vi "1SDI_State_v00.vi"(4 "BS Hold Pulse":bool, 6 "\"I too high?\"":T6, 11 "Control Cavity Cluster":T11={"Control EPR"={"Lock"=FALSE, "Hold"=FALSE, "P Gain"=0, "P BS"=-5, "I Gain"=0, "I BS"=-10, "I2 G"=0, "I2 BS"=-26, "Scan Amp"=0, "Scan Off"=0, "Scan FS"=0, "SFS BS"=0, "I Max value"=10000, "I2 Max value"=10000, "Scope.Offset"=0, "Trigger Direction"=enum."either", "Scan-PII thresh"=0}, "Control HD A"={"Lock"=FALSE, "Hold"=FALSE, "P Gain"=0, "P BS"=-5, "I Gain"=0, "I BS"=-10, "I2 G"=0, "I2 BS"=-26, "Scan Amp"=0, "Scan Off"=0, "Scan FS"=0, "SFS BS"=0, "I Max value"=10000, "I2 Max value"=10000, "Scope.Offset"=0, "Trigger Direction"=enum."either", "Scan-PII thresh"=0}, "Control HD B"={"Lock"=FALSE, "Hold"=FALSE, "P Gain"=0, "P BS"=-5, "I Gain"=0, "I BS"=-10, "I2 G"=0, "I2 BS"=-26, "Scan Amp"=0, "Scan Off"=0, "Scan FS"=0, "SFS BS"=0, "I Max value"=10000, "I2 Max value"=10000, "Scope.Offset"=0, "Trigger Direction"=enum."either", "Scan-PII thresh"=0}, "Max"={"Max EPR"=0, "Max HD A"=0, "Max HD B"=0}, "Min"={"Min EPR"=0, "Min HD A"=0, "Min HD B"=0}, "Lock Threshold"={"EPR"=0, "HD A"=0, "HD B"=0}, "Re-Scan Threshold"={"EPR"=0, "HD A"=0, "HD B"=0}, "Lock Point?"={"EPR"=FALSE, "HD A"=FALSE, "HD B"=FALSE}, "Re-scan?"={"EPR"=FALSE, "HD A"=FALSE, "HD B"=FALSE}, "Lock pressed? (-1)"={"EPR"=FALSE, "HD A"=FALSE, "HD B"=FALSE}, "Cavity Errors"={"EPR"=0, "HD A"=0, "HD B"=0}, "State (-1)"={"EPR"=enum."Safe", "HD A"=enum."Safe", "HD B"=enum."Safe"}, "Safety First"={"lim reset"=FALSE, "no limit"=FALSE, "pos slew rate * dt"=0, "neg slew rate * dt"=0, "Hold All"=FALSE, "Count(Ticks)"=0}}) -> (3 "PII Scan State Errors":T8={"Control EPR"={"Lock"=FALSE, "Hold"=FALSE, "P Gain"=3, "P BS"=0, "I Gain"=0, "I BS"=-10, "I2 G"=0, "I2 BS"=-26, "Scan Amp"=0, "Scan Off"=0, "Scan FS"=0, "SFS BS"=0, "I Max value"=10000, "I2 Max value"=10000, "Scope.Offset"=0, "Trigger Direction"=enum."either", "Scan-PII thresh"=0}, "Control HD A"={"Lock"=FALSE, "Hold"=FALSE, "P Gain"=0, "P BS"=-5, "I Gain"=0, "I BS"=-10, "I2 G"=0, "I2 BS"=-26, "Scan Amp"=0, "Scan Off"=0, "Scan FS"=0, "SFS BS"=0, "I Max value"=10000, "I2 Max value"=10000, "Scope.Offset"=0, "Trigger Direction"=enum."either", "Scan-PII thresh"=0}, "Control HD B"={"Lock"=FALSE, "Hold"=FALSE, "P Gain"=0, "P BS"=-5, "I Gain"=0, "I BS"=-10, "I2 G"=0, "I2 BS"=-26, "Scan Amp"=0, "Scan Off"=0, "Scan FS"=0, "SFS BS"=0, "I Max value"=10000, "I2 Max value"=10000, "Scope.Offset"=0, "Trigger Direction"=enum."either", "Scan-PII thresh"=0}, "Error Signals"={"EPR"=0, "HD A"=0, "HD B"=0}, "State"={"EPR"=enum."Safe", "HD A"=enum."Safe", "HD B"=enum."Safe"}}, 5 "MaxMin":T1)   [LabVIEW 2011]
doc: "The state of the output is decided here. There are four possible states: 1) Safe - zeros; 2) Hold - constant output of last value; 3) Scan - saw tooth at low frequency 4) Lock - PII output."
uses:
  Strict Type Defs/1SDI State.ctl
  Strict Type Defs/1SDI PII Scan State.ctl
  Strict Type Defs/PII individual.ctl
  Strict Type Defs/Error Signals 1SDI.ctl
  Strict Type Defs/1SDI Lock Point.ctl
  Strict Type Defs/1SDI Control Cluster.ctl
  Strict Type Defs/1SDI Max.ctl
  Strict Type Defs/1SDI Min.ctl
  Strict Type Defs/Lock Thresh 1SDI.ctl
  Strict Type Defs/Safety First.ctl
  Strict Type Defs/1SDI MaxMin.ctl
  Strict Type Defs/1SDI Reset MaxMin.ctl
panel:
  in  "MaxMin typedef":T1
  in  "Lock?":T6
  in  "PII Scan State":T8={"Control EPR"={"Lock"=FALSE, "Hold"=FALSE, "P Gain"=3, "P BS"=0, "I Gain"=0, "I BS"=-10, "I2 G"=0, "I2 BS"=-26, "Scan Amp"=0, "Scan Off"=0, "Scan FS"=0, "SFS BS"=0, "I Max value"=10000, "I2 Max value"=10000, "Scope.Offset"=0, "Trigger Direction"=enum."either", "Scan-PII thresh"=0}, "Control HD A"={"Lock"=FALSE, "Hold"=FALSE, "P Gain"=0, "P BS"=-5, "I Gain"=0, "I BS"=-10, "I2 G"=0, "I2 BS"=-26, "Scan Amp"=0, "Scan Off"=0, "Scan FS"=0, "SFS BS"=0, "I Max value"=10000, "I2 Max value"=10000, "Scope.Offset"=0, "Trigger Direction"=enum."either", "Scan-PII thresh"=0}, "Control HD B"={"Lock"=FALSE, "Hold"=FALSE, "P Gain"=0, "P BS"=-5, "I Gain"=0, "I BS"=-10, "I2 G"=0, "I2 BS"=-26, "Scan Amp"=0, "Scan Off"=0, "Scan FS"=0, "SFS BS"=0, "I Max value"=10000, "I2 Max value"=10000, "Scope.Offset"=0, "Trigger Direction"=enum."either", "Scan-PII thresh"=0}, "Error Signals"={"EPR"=0, "HD A"=0, "HD B"=0}, "State"={"EPR"=enum."Safe", "HD A"=enum."Safe", "HD B"=enum."Safe"}}
  in  "State":T2
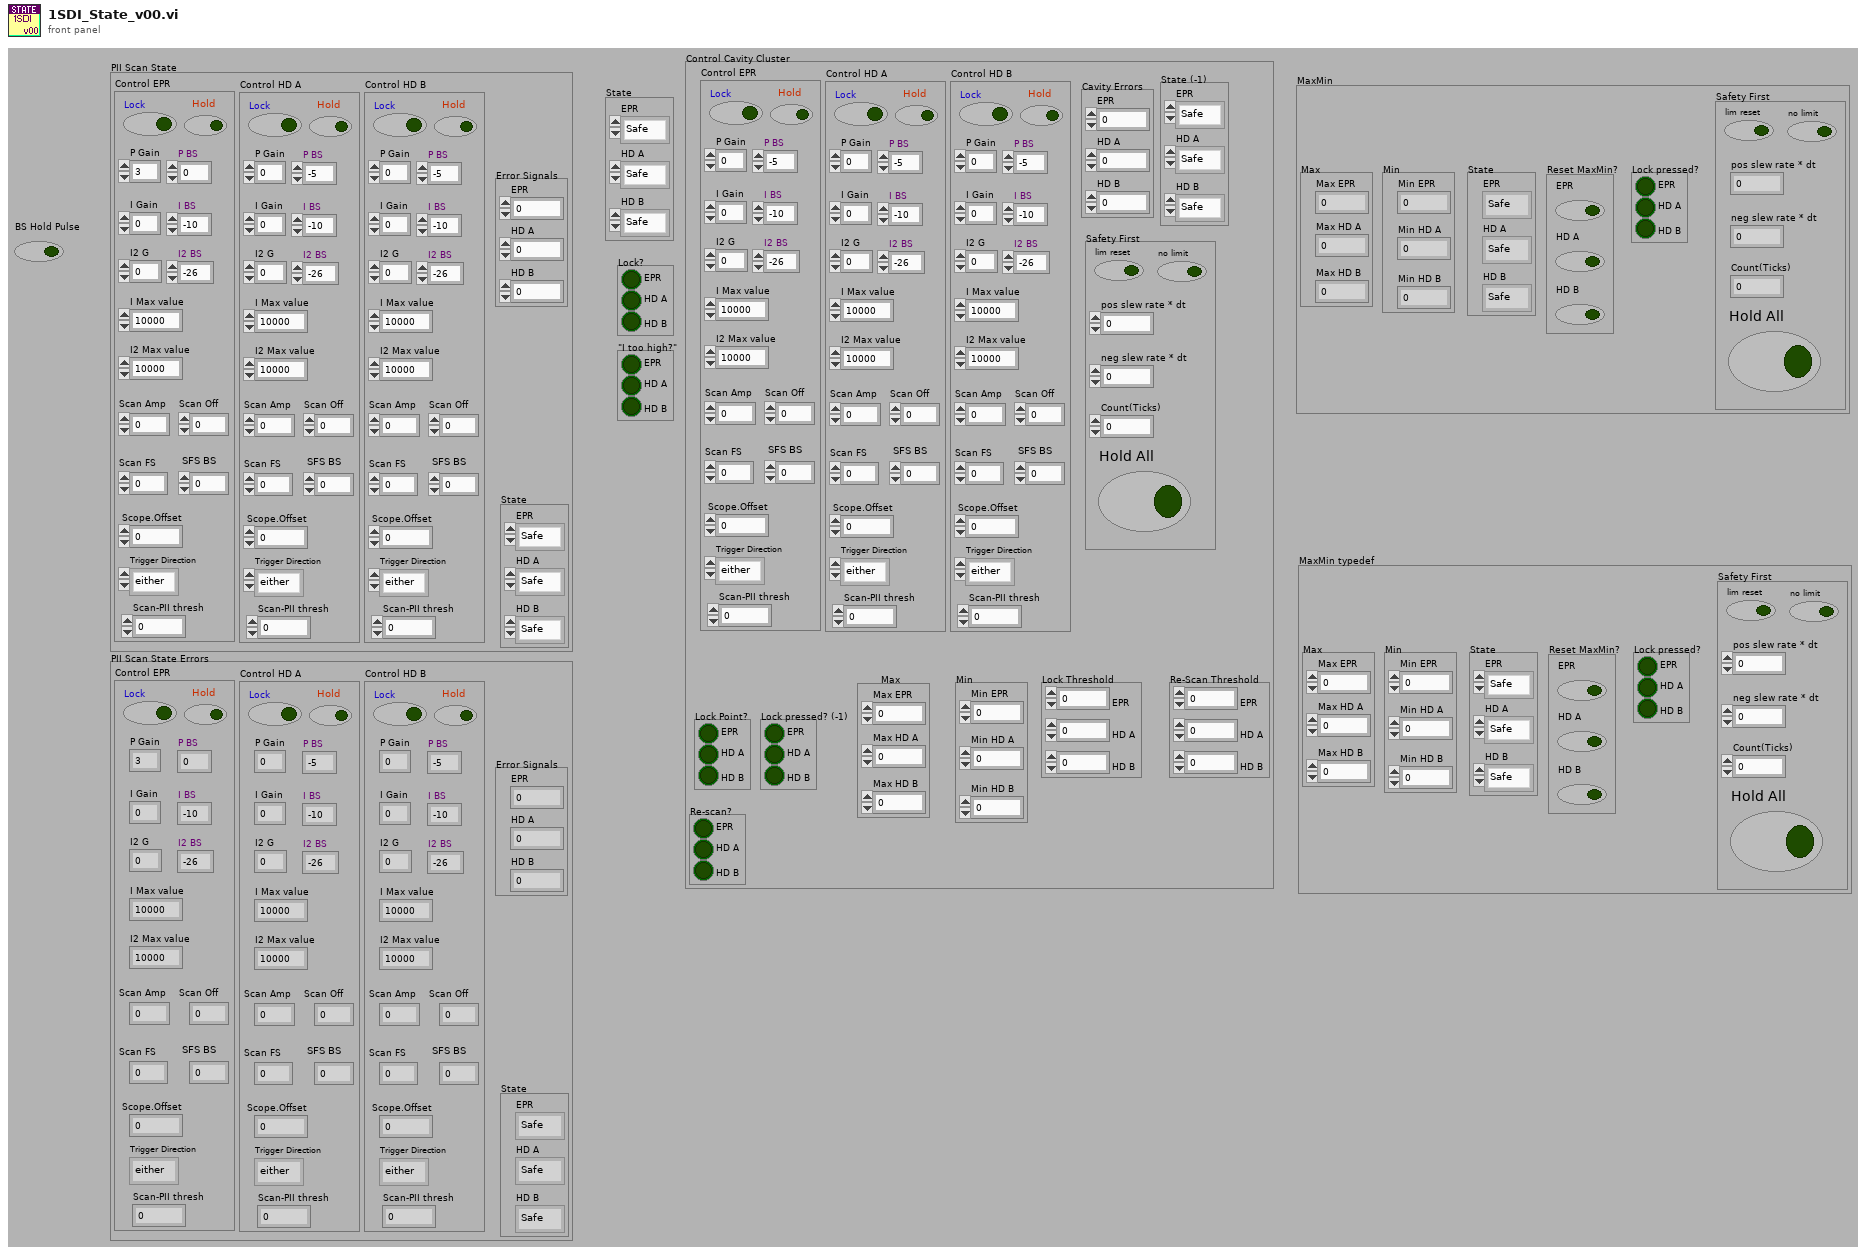
[diagram p1: front panel]
types:
  T1 = typedef "1SDI MaxMin.ctl" = cluster{"State":T2, "Reset MaxMin?":T3, "Max":T4, "Min":T5, "Lock pressed?":T6, "Safety First":T7}
  T2 = typedef "1SDI State.ctl" = cluster{"EPR":enum16{"Safe", "Hold", "Scan", "Lock"}, "HD A":enum16{"Safe", "Hold", "Scan", "Lock"}, "HD B":enum16{"Safe", "Hold", "Scan", "Lock"}}
  T3 = typedef "1SDI Reset MaxMin.ctl" = cluster{"EPR":bool, "HD A":bool, "HD B":bool}
  T4 = typedef "1SDI Max.ctl" = cluster{"Max EPR":i16, "Max HD A":i16, "Max HD B":i16}
  T5 = typedef "1SDI Min.ctl" = cluster{"Min EPR":i16, "Min HD A":i16, "Min HD B":i16}
  T6 = typedef "1SDI Lock Point.ctl" = cluster{"EPR":bool, "HD A":bool, "HD B":bool}
  T7 = typedef "Safety First.ctl" = cluster{"lim reset":bool, "no limit":bool, "pos slew rate * dt":i16, "neg slew rate * dt":i16, "Hold All":bool, "Count(Ticks)":u32}
  T8 = typedef "1SDI PII Scan State.ctl" = cluster{"Control EPR":T9, "Control HD A":T9, "Control HD B":T9, "Error Signals":T10, "State":T2}
  T9 = typedef "PII individual.ctl" = cluster{"Lock":bool, "Hold":bool, "P Gain":i32, "P BS":i16, "I Gain":i32, "I BS":i16, "I2 G":i32, "I2 BS":i16, "Scan Amp":i16, "Scan Off":i16, "Scan FS":u16, "SFS BS":i16, "I Max value":i32, "I2 Max value":i32, "Scope.Offset":i16, "Trigger Direction":enum8{"either", "minus-plus", "plus-minus"}, "Scan-PII thresh":i16}
  T10 = typedef "Error Signals 1SDI.ctl" = cluster{"EPR":i16, "HD A":i16, "HD B":i16}
  T11 = typedef "1SDI Control Cluster.ctl" = cluster{"Control EPR":T9, "Control HD A":T9, "Control HD B":T9, "Max":T4, "Min":T5, "Lock Threshold":T12, "Re-Scan Threshold":T12, "Lock Point?":T6, "Re-scan?":T6, "Lock pressed? (-1)":T6, "Cavity Errors":T10, "State (-1)":T2, "Safety First":T7}
  T12 = typedef "Lock Thresh 1SDI.ctl" = cluster{"EPR":i16, "HD A":i16, "HD B":i16}
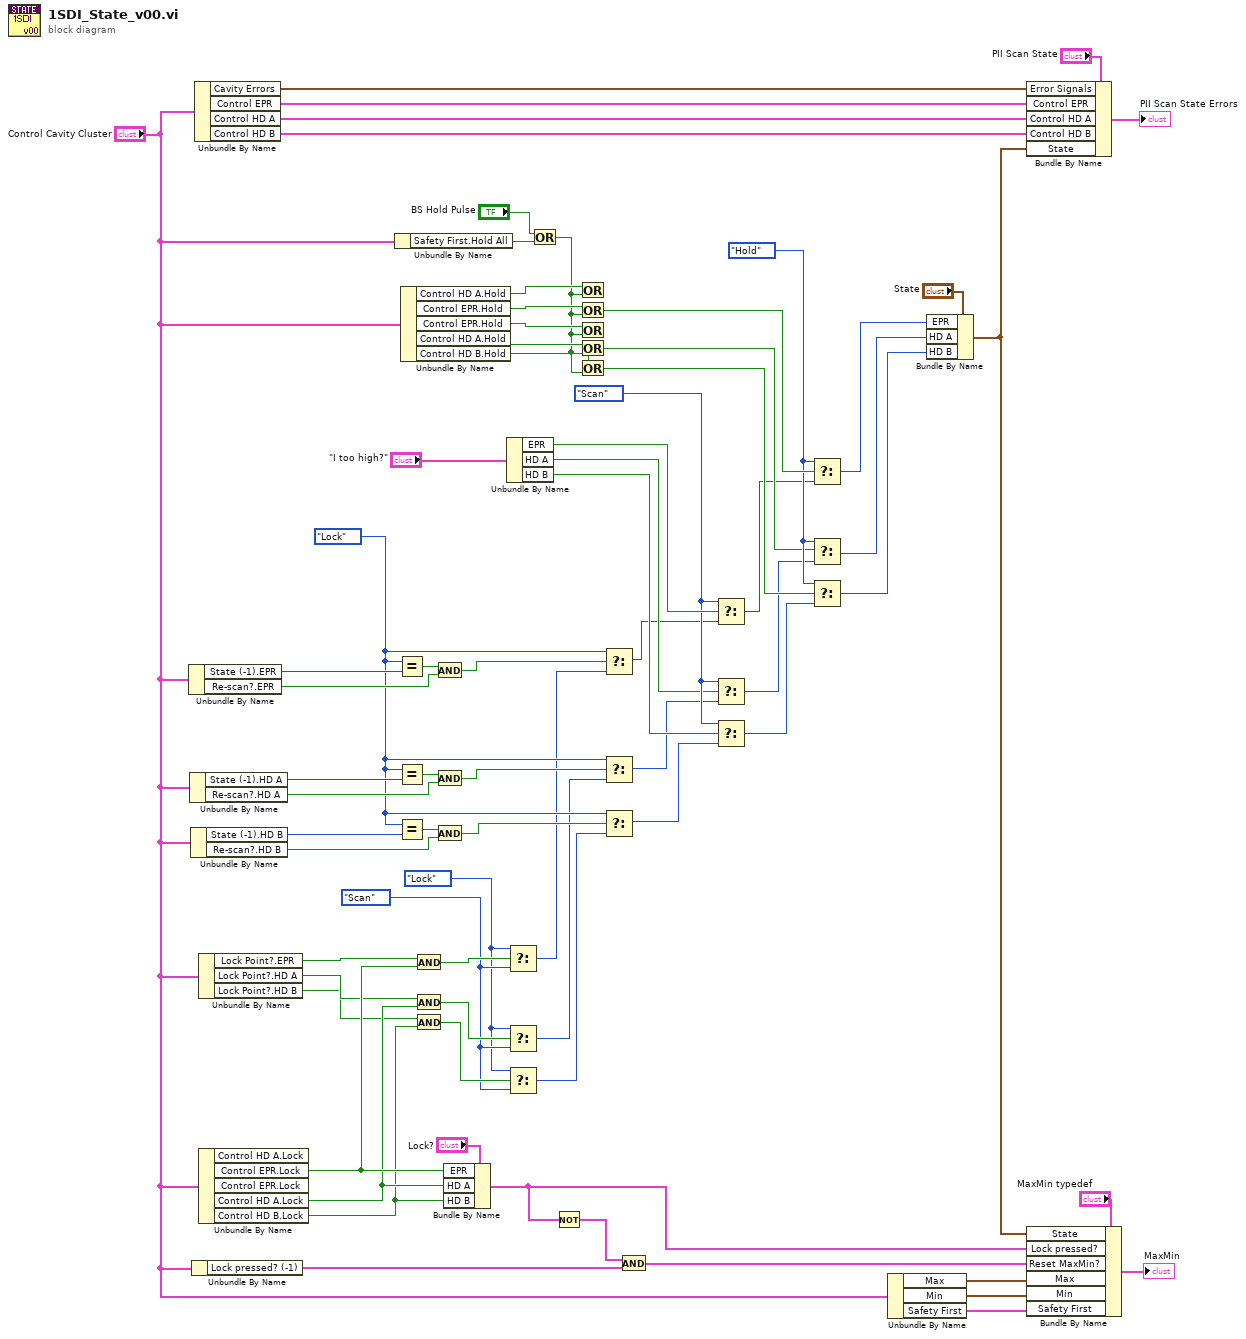
[diagram p0: block diagram]
diagram:
  w24 = enum16{"Safe", "Hold", "Scan", "Lock"}."Scan" ("State")
  w35 = enum16{"Safe", "Hold", "Scan", "Lock"}."Lock" ("y")
  w25 = enum16{"Safe", "Hold", "Scan", "Lock"}."Hold" ("State")
  w27 = enum16{"Safe", "Hold", "Scan", "Lock"}."Scan" ("State")
  w26 = enum16{"Safe", "Hold", "Scan", "Lock"}."Lock" ("State")
  n1 = Unbundle By Name("Control Cavity Cluster") -> ("State (-1).EPR"=w48:enum16{"Safe", "Hold", "Scan", "Lock"}, "Re-scan?.EPR"=w67:bool)
  n2 = Unbundle By Name("Control Cavity Cluster") -> ("State (-1).HD A"=w43:enum16{"Safe", "Hold", "Scan", "Lock"}, "Re-scan?.HD A"=w39:bool)
  n3 = Unbundle By Name("Control Cavity Cluster") -> ("State (-1).HD B"=w42:enum16{"Safe", "Hold", "Scan", "Lock"}, "Re-scan?.HD B"=w38:bool)
  n4 = Unbundle By Name("Control Cavity Cluster") -> ("Lock pressed? (-1)"=w59:T6)
  n5 = Unbundle By Name("Control Cavity Cluster") -> ("Cavity Errors"=w63:T10, "Control EPR"=w62:T9, "Control HD A"=w33:T9, "Control HD B"=w32:T9)
  n6 = Unbundle By Name("Control Cavity Cluster") -> ("Lock Point?.EPR"=w50:bool, "Lock Point?.HD A"=w19:bool, "Lock Point?.HD B"=w17:bool)
  n7 = Unbundle By Name("Control Cavity Cluster") -> ("Control EPR.Lock"=w49:bool, "Control HD A.Lock"=w18:bool, "Control HD B.Lock"=w16:bool)  [unwired: 2 out]
  n8 = Unbundle By Name("Control Cavity Cluster") -> ("Safety First.Hold All"=w9:bool)
  n9 = Equal?(x=w35, y=w48) -> (x = y?=w66:bool)
  n10 = Equal?(x=w35, y=w43) -> (x = y?=w40:bool)
  n11 = Equal?(x=w35, y=w42) -> (x = y?=w37:bool)
  n12 = Unbundle By Name("Control Cavity Cluster") -> ("Control HD A.Hold"=w53:bool, "Control EPR.Hold"=w52:bool, "Control EPR.Hold"=w51:bool, "Control HD A.Hold"=w31:bool, "Control HD B.Hold"=w30:bool)
  n13 = And(x=w50, y=w49) -> (x .and. y?=w70:bool)
  n14 = And(x=w19, y=w18) -> (x .and. y?=w29:bool)
  n15 = And(x=w17, y=w16) -> (x .and. y?=w28:bool)
  n16 = And(x=w66, y=w67) -> (x .and. y?=w65:bool)
  n17 = And(x=w40, y=w39) -> (x .and. y?=w41:bool)
  n18 = And(x=w37, y=w38) -> (x .and. y?=w36:bool)
  n19 = Bundle By Name(cluster="Lock?", "EPR"=w49, "HD A"=w18, "HD B"=w16) -> (w45:T6)
  n20 = Unbundle By Name("\"I too high?\"") -> ("EPR"=w55:bool, "HD A"=w21:bool, "HD B"=w20:bool)
  n21 = Select(t=w26, s=w70, f=w27) -> (s? t:f=w15:enum16{"Safe", "Hold", "Scan", "Lock"})
  n22 = Select(t=w26, s=w29, f=w27) -> (s? t:f=w14:enum16{"Safe", "Hold", "Scan", "Lock"})
  n23 = Select(t=w26, s=w28, f=w27) -> (s? t:f=w13:enum16{"Safe", "Hold", "Scan", "Lock"})
  n24 = Or(x="BS Hold Pulse", y=w9) -> (x .or. y?=w7:bool)
  n25 = Not(x=w45) -> (.not. x?=w64:T6)
  n26 = Or(x=w53, y=w7) -> ()  [unwired: 1 out]
  n27 = Or(x=w52, y=w7) -> (x .or. y?=w68:bool)
  n28 = Or(x=w51, y=w7) -> ()  [unwired: 1 out]
  n29 = Or(x=w31, y=w7) -> (x .or. y?=w23:bool)
  n30 = Or(x=w30, y=w7) -> (x .or. y?=w22:bool)
  n31 = Select(t=w35, s=w65, f=w15) -> (s? t:f=w12:enum16{"Safe", "Hold", "Scan", "Lock"})
  n32 = Select(t=w35, s=w41, f=w14) -> (s? t:f=w11:enum16{"Safe", "Hold", "Scan", "Lock"})
  n33 = Select(t=w35, s=w36, f=w13) -> (s? t:f=w10:enum16{"Safe", "Hold", "Scan", "Lock"})
  n34 = And(x=w64, y=w59) -> (x .and. y?=w57:T6)
  n35 = Select(t=w24, s=w55, f=w12) -> (s? t:f=w6:enum16{"Safe", "Hold", "Scan", "Lock"})
  n36 = Select(t=w24, s=w21, f=w11) -> (s? t:f=w5:enum16{"Safe", "Hold", "Scan", "Lock"})
  n37 = Select(t=w24, s=w20, f=w10) -> (s? t:f=w4:enum16{"Safe", "Hold", "Scan", "Lock"})
  n38 = Select(t=w25, s=w68, f=w6) -> (s? t:f=w3:enum16{"Safe", "Hold", "Scan", "Lock"})
  n39 = Select(t=w25, s=w23, f=w5) -> (s? t:f=w2:enum16{"Safe", "Hold", "Scan", "Lock"})
  n40 = Select(t=w25, s=w22, f=w4) -> (s? t:f=w1:enum16{"Safe", "Hold", "Scan", "Lock"})
  n41 = Unbundle By Name("Control Cavity Cluster") -> ("Max"=w47:T4, "Min"=w46:T5, "Safety First"=w44:T7)
  n42 = Bundle By Name(cluster="State", "EPR"=w3, "HD A"=w2, "HD B"=w1) -> (w56:T2)
  n43 = Bundle By Name(cluster="PII Scan State", "Error Signals"=w63, "Control EPR"=w62, "Control HD A"=w33, "Control HD B"=w32, "State"=w56) -> (→"PII Scan State Errors":T8)
  n44 = Bundle By Name(cluster="MaxMin typedef", "State"=w56, "Lock pressed?"=w45, "Reset MaxMin?"=w57, "Max"=w47, "Min"=w46, "Safety First"=w44) -> (→"MaxMin":T1)
